vi "EdgeDetect.vi"() -> ()   [LabVIEW 2022 SP3]
panel:
  out "觸發計數":i32
  in  "stop":bool
  in  "硬體外部輸入...":bool
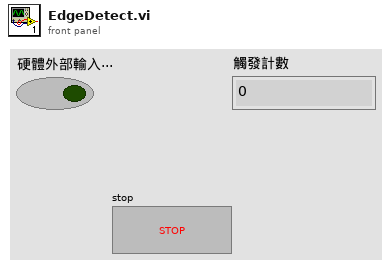
[diagram p1: front panel]
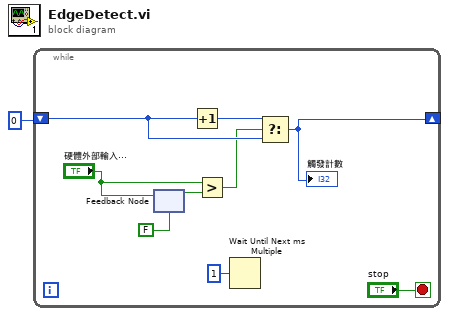
[diagram p0: block diagram]
diagram:
  n1 = while {
    shift-right: [w8] -> _
    shift-left: 0 -> [w9]
    stop <- "stop" stop-if-true
    n2 = feedback-in #1("硬體外部輸入...") -> ()
    n3 = feedback #1(FALSE) -> (w4:bool)
    n4 = Increment(x=w9) -> (x+1=w10:i32)
    n5 = Greater?(x="硬體外部輸入...", y=w4) -> (0:w2:bool)
    n6 = Wait Until Next ms Multiple(millisecond multiple=u32 1) -> ()  [unwired: 1 out]
    n7 = Select(t=w10, s=w2, f=w9) -> (s? t:f=w8:i32)
    "觸發計數" <- w8
  }
